vi "LowPassForce.vi"(0 "reference in":refnum<class "PassSkill.lvclass">, 5 "error in (no error)":errorcluster) -> (14 "reference out":refnum<class "PassSkill.lvclass">, 19 "error out":errorcluster)   [LabVIEW 2023, in "PassSkill.lvclass"]
uses:
  PassSkill.lvclass
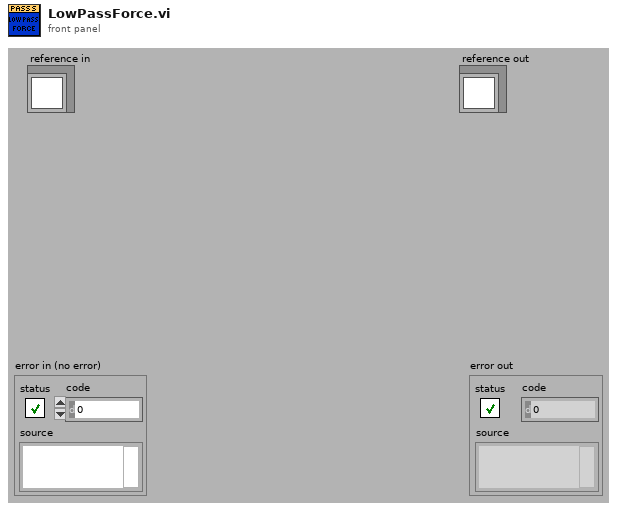
[diagram p1: front panel]
types:
  T1 = typedef "PassSkill.lvclass/ObjectAttributes.ctl" = cluster{"None":bool}
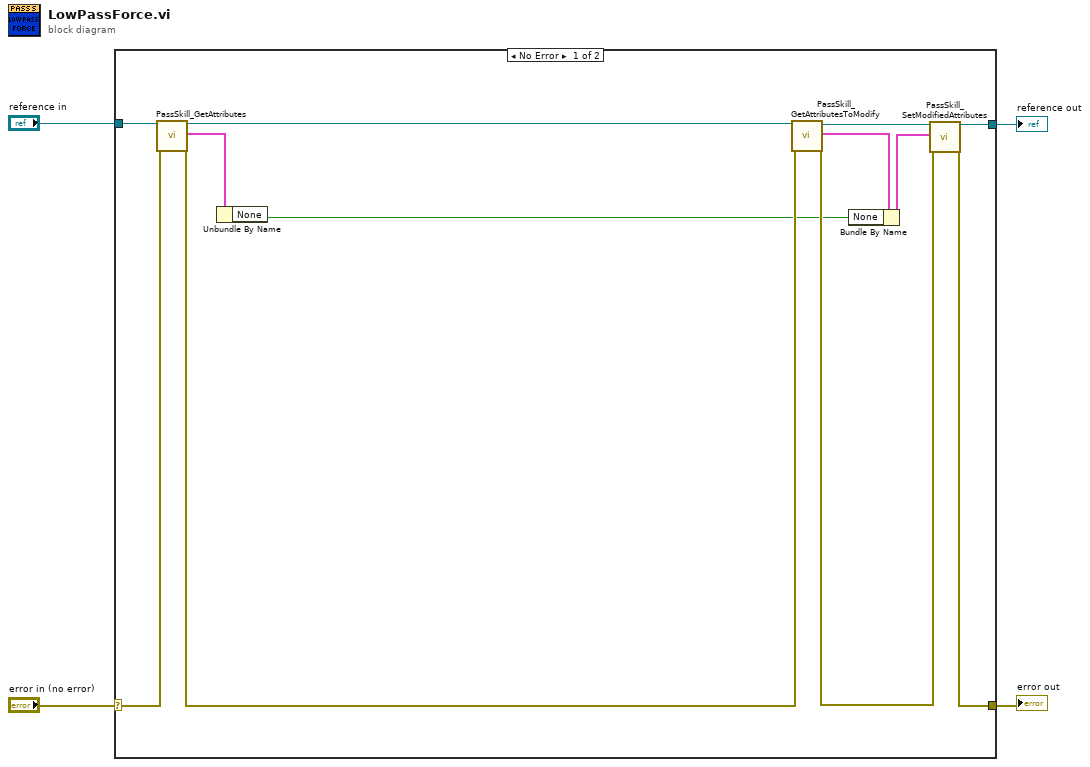
[diagram p0: block diagram]
diagram:
  n1 = case shown="No Error" "error in (no error)" {
    selector: "error in (no error)" -> [w9 w18]
    tunnel: [w13 w18] -> w3
    tunnel: [w12 w17] -> w1
    tunnel: "reference in" -> [w10 w17]
    frame No Error {
      n2 = call "PassSkill_GetAttributes.vi"("reference in"=w10, "error in (no error)"=w9) -> ("reference out"=w7:refnum<class "PassSkill.lvclass">, "Attributes"=w6:T1, "error out"=w8:errorcluster)  [unwired: 14 in, 1 out]
      n3 = Unbundle By Name(w6) -> ("None"=w5:bool)
      n4 = call "PassSkill_GetAttributesToModify.vi"("reference in"=w7, "error in (no error)"=w8) -> ("reference out"=w14:refnum<class "PassSkill.lvclass">, "Attributes"=w16:T1, "error out"=w11:errorcluster)  [unwired: 14 in, 1 out]
      n5 = Bundle By Name(cluster=w16, "None"=w5) -> (w15:T1)
      n6 = call "PassSkill_SetModifiedAttributes.vi"("reference in"=w14, "Attributes"=w15, "error in (no error)"=w11) -> ("reference out"=w12:refnum<class "PassSkill.lvclass">, "error out"=w13:errorcluster)  [unwired: 15 in]
    }
    frame Error {
    }
  }
  "error out" <- w3
  "reference out" <- w1
